vi "ConfigureMarkerFrequencyCounter.vi"(8 "error in (no error)":errorcluster, 11 "Keysight44xx in":refnum<class "Keysight44xx.lvclass">) -> (0 "error out":errorcluster, 3 "Keysight44xx out":refnum<class "Keysight44xx.lvclass">)   [LabVIEW 2018, in "SpecAnPlugins.lvlib" / "Keysight44xx.lvclass"]
doc: "This VI sets the marker frequency counter resolution and turns the marker frequency counter on/off."
uses:
  Keysight44xx.lvclass
  C:/Users/ico/Documents/Projects/NistPluggableModules/SpecAn/SpecAnPlugins/SpecAnBaseClass/SpecAnBase.lvclass
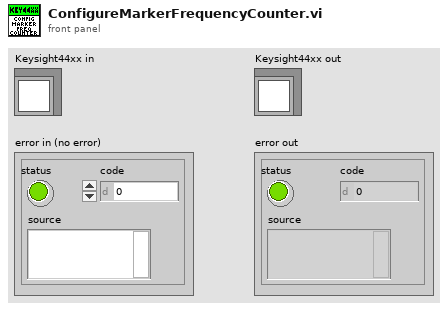
[diagram p1: front panel]
types:
  T1 = typedef "SpecAnPlugins.lvlib/SpecAnBase.lvclass/Acquisition.ctl" = cluster{"Handle":string, "Connected":bool, "Enabled":bool, "SweepModeContinuous":bool, "NumberOfSweeps":i32, "DetectorTypeAuto":bool, "DetectorType":i32, "VerticalScale":i32, "MaximumTime(seconds)":dbl}
  T2 = typedef "SpecAnPlugins.lvlib/SpecAnBase.lvclass/Markers.ctl" = cluster{"MarkerEnabled":bool, "MarkerThreshold":dbl, "PeakExcursion":dbl, "SignalTrackEnabled":bool, "MarkerPosition":dbl, "Instrument Setting (Frequency Center)":i32, "Marker search (Minimum)":i32, "ActiveMarker":string, "MarkerFrequencyCounter":bool, "FrequencyCounterResolution":dbl}
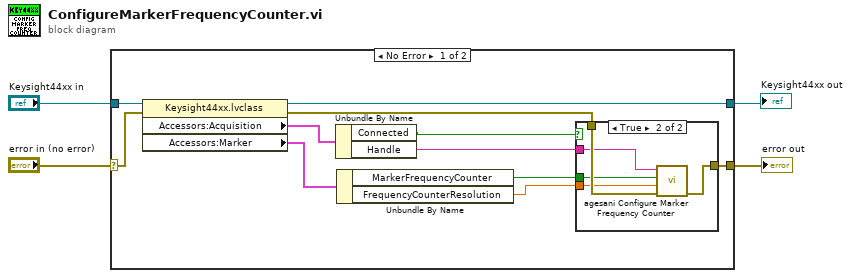
[diagram p0: block diagram]
diagram:
  n1 = case shown="No Error" "error in (no error)" {
    selector: "error in (no error)" -> [w13 w23]
    tunnel: "Keysight44xx in" -> [w15 w22]
    tunnel: [w14 w22] -> w3
    tunnel: [w6 w23] -> w1
    frame No Error {
      n2 = property class="Keysight44xx.lvclass"(reference=w15, error in=w13) -> (reference out=w14:refnum<class "Keysight44xx.lvclass">, error out=w10:errorcluster, "Accessors:Acquisition"=w12:T1, "Accessors:Marker"=w11:T2)
      n3 = Unbundle By Name(w12) -> ("Connected"=w5:bool, "Handle"=w9:string)
      n4 = Unbundle By Name(w11) -> ("MarkerFrequencyCounter"=w8:bool, "FrequencyCounterResolution"=w7:dbl)
      n5 = case shown="True" w5 {
        tunnel: w10 -> [w16 w21]
        tunnel: w9 -> [_ w20]
        tunnel: w8 -> [_ w19]
        tunnel: w7 -> [_ w18]
        tunnel: [w16 w17] -> w6
        frame False {
        }
        frame True {
          n6 = call <instrlib>:"agesani Configure Marker Frequency Counter.vi"("error in (no error)"=w21, "frequency counter resolution (1.0e3)"=w18, "marker frequency counter (Off)"=w19, "instrument handle"=w20) -> ("error out"=w17:errorcluster)  [unwired: 6 in, 1 out]
        }
      }
    }
    frame Error {
    }
  }
  "error out" <- w1
  "Keysight44xx out" <- w3
